vi "TPNT_ModifyDevice.vi"(8 "error in (no error)":errorcluster, 10 "arguments":string, 11 "Object Refnum In":T1) -> (0 "error out":errorcluster, 3 "Data Refnum out":T1)   [LabVIEW 2016]
uses:
  TPNT_Refnum.ctl
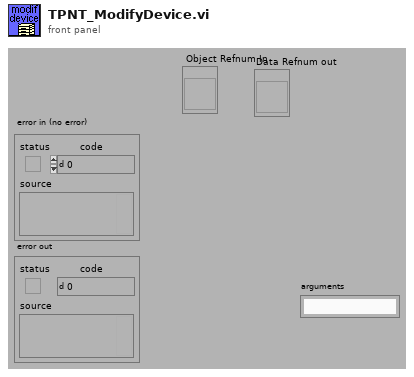
[diagram p1: front panel]
types:
  T1 = typedef "TPNT_Refnum.ctl" = refnum<vi>
  T2 = typedef "TPNT_DeviceTPs.ctl" = cluster{"device":string, "devupdate":dbl, "next_update":u32, "devinterface":string, "TPs":T3[], "Alarms":bool, "monitor":bool, "log sep":string}
  T3 = typedef "TPNT_TP.ctl" = cluster{"name":string, "type":string, "algor":string[], "update_rate":sgl, "Limits":T4, "Samples":T5, "next_update":u32, "Status":string, "monitor":bool, "error":bool, "Log":T6, "permissions":string, "ID":string}
  T4 = typedef "TPNT_Limits.ctl" = cluster{"Alarm Type":string, "Lower ":dbl, "Upper":dbl, "Nominal":dbl, "outrange":bool, "Check":bool, "latch":bool, "level":string}
  T5 = typedef "TPNT_Samples.ctl" = cluster{"samples":i32, "counter":i32, "Values":dbl[], "Current Value":string, "filter":string, "precision":u8}
  T6 = typedef "TPNT_Log.ctl" = cluster{"log":bool, "file":path, "type":string, "format":string, "updaterate":dbl, "nex_update":u32, "mode":string}
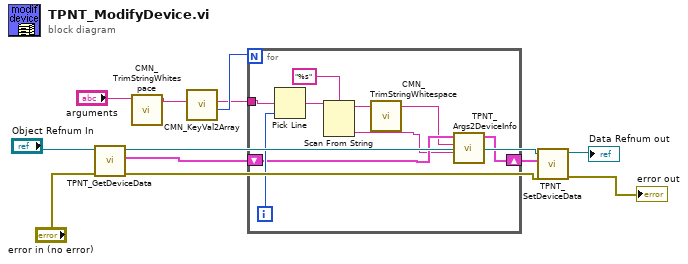
[diagram p0: block diagram]
diagram:
  n1 = call "TPNT_GetDeviceData.vi"("error in (no error)"="error in (no error)", "Object Refnum In"="Object Refnum In") -> ("error out"=w2:errorcluster, "Object Data Out"=w4:T2, "Data Refnum out"=w1:T1)  [unwired: 7 out]
  n2 = call "CMN_TrimStringWhitespace.vi"("string"="arguments") -> ("trimmed string"=w7:string)  [unwired: 1 in, 8 out]
  n3 = call "CMN_KeyVal2Array.vi"("command in"=w7) -> ("number of commands"=w10:i32, "commands out"=w9:string)  [unwired: 2 in, 6 out]
  n4 = for {
    N: w10 -> [_]
    tunnel: w9 -> [w21]
    shift-right: [w15] -> w6
    shift-left: w4 -> [w16]
    i -> [w20]
    n5 = Pick Line(multi-line string=w21, line index=w20) -> (output string=w19:string)  [unwired: 1 out]
    n6 = Scan From String(format string="%s", input string=w19) -> (remaining string=w17:string, output 1=w13:string)  [unwired: 2 in, 3 out]
    n7 = call "CMN_TrimStringWhitespace.vi"("string"=w17) -> ("trimmed string"=w14:string)  [unwired: 1 in, 8 out]
    n8 = call "TPNT_Args2DeviceInfo.vi"("key"=w13, "value"=w14, "Device IN"=w16) -> ("Device OUT"=w15:T2)  [unwired: 8 out]
  }
  n9 = call "TPNT_SetDeviceData.vi"("error in (no error)"=w2, "Object Data In"=w6, "Object Refnum In"=w1) -> ("error out"=→"error out":errorcluster, "Data Refnum out"=→"Data Refnum out":T1)  [unwired: 7 out]
